vi "AddChannel.vi"(0 "VIRef":refnum<vi>[](array[refnum]), 1 "Name":string="172.16.21.19", 3 "SetCurrent":dbl format="%#.2g", 5 "ADRESS":string[](array[string]), 7 "error in (no error)":errorcluster, 9 "NAME":string[](array[string]), 11 "Address":string="172.16.21.19", 12 "SetVoltage":dbl format="%#.2g") -> (4 "NumRows":i32, 6 "NAMEOut":string[](array[string]), 8 "error out":errorcluster, 10 "ADRESSOut":string[](array[string]), 15 "VIRefOut":refnum<vi>[](array[refnum]))   [LabVIEW 2013]
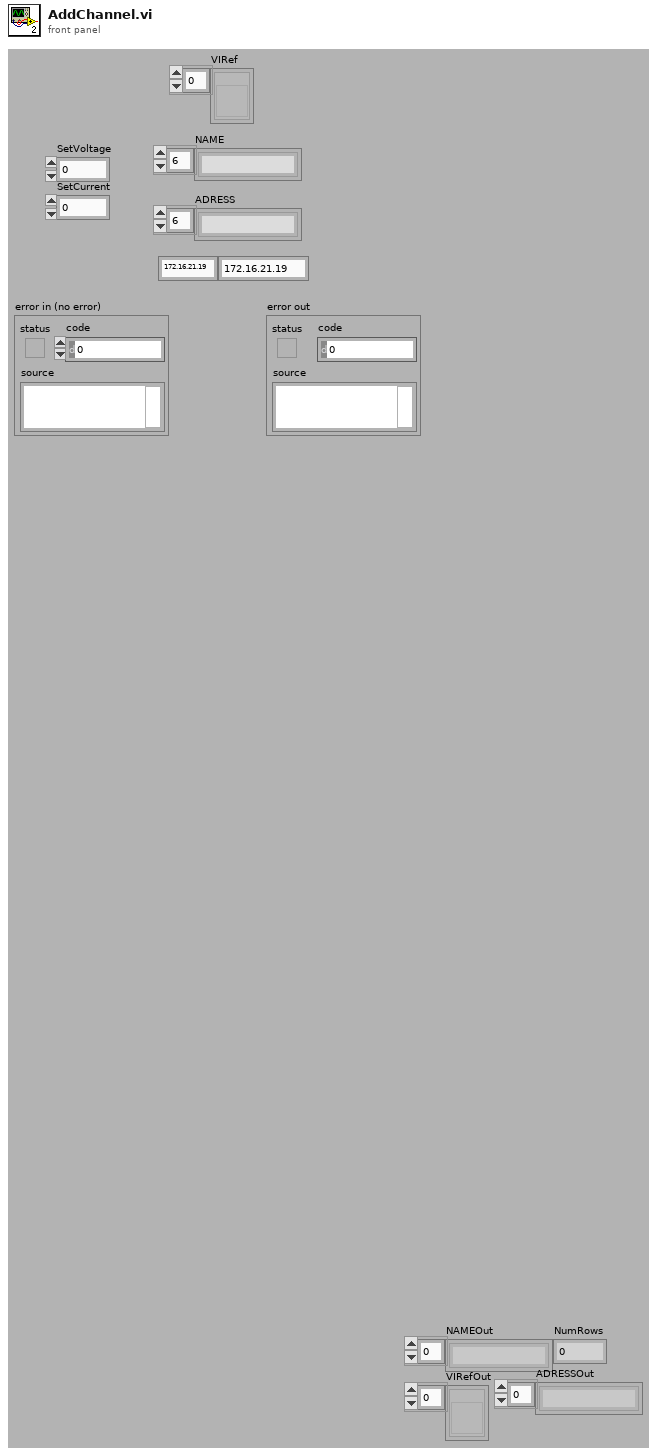
[diagram p1: front panel]
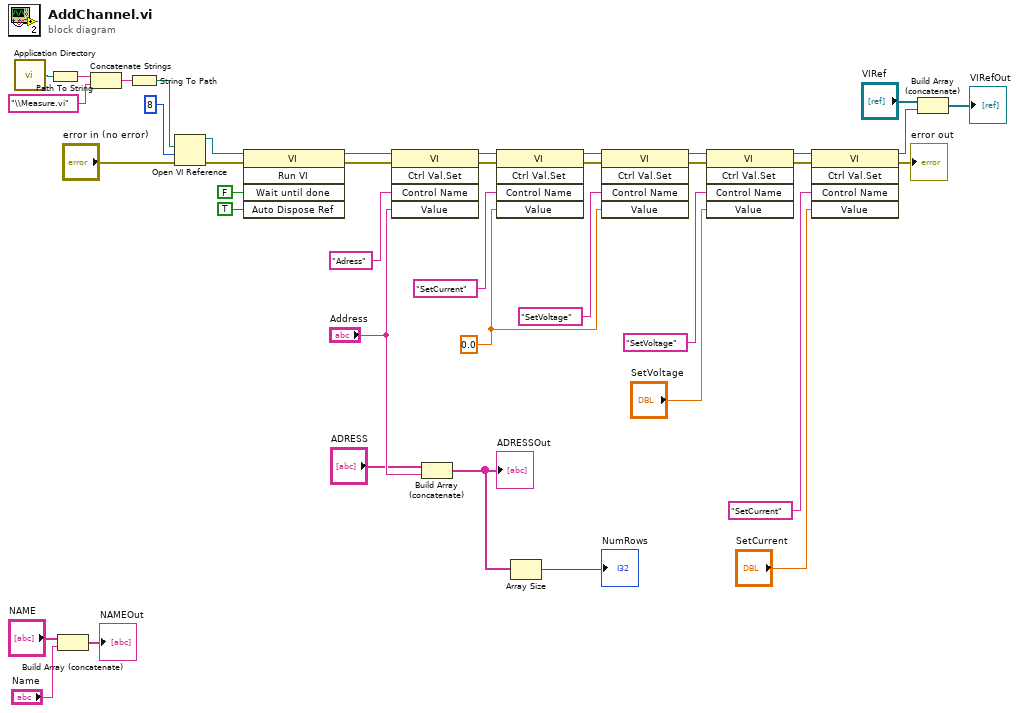
[diagram p0: block diagram]
diagram:
  w20 = 0.0 ("SetCurrent")
  n1 = call <vilib>:"Application Directory.vi"() -> ("Application Directory"=w1:path)
  n2 = Path To String(path=w1) -> (string=w5:string)
  n3 = Build Array (concatenate)("NAME", "Name") -> (→"NAMEOut":string[])
  n4 = Concatenate Strings(w5, "\\Measure.vi" ("string")) -> (w3:string)
  n5 = String To Path(string=w3) -> (path=w2:path)
  n6 = Open VI Reference(vi path=w2, options=8, error in (no error)="error in (no error)") -> (vi reference=w36:refnum<vi>, error out=w39:errorcluster)  [unwired: 1 in, 2 out]
  n7 = invoke class="VI" method="Run VI"(reference=w36, error in=w39, "Wait until done"=FALSE ("Wait Until Done"), "Auto Dispose Ref"=TRUE ("Auto Dispose Reference")) -> (reference out=w33:refnum<vi>, error out=w23:errorcluster)  [unwired: 1 in, 3 out]
  n8 = invoke class="VI" method="Ctrl Val.Set"(reference=w33, error in=w23, "Control Name"="Adress", "Value"="Address") -> (reference out=w25:refnum<vi>, error out=w22:errorcluster)  [unwired: 1 in, 3 out]
  n9 = Build Array (concatenate)("ADRESS", "Address") -> (w31:string[])
  "ADRESSOut" <- w31
  n10 = invoke class="VI" method="Ctrl Val.Set"(reference=w25, error in=w22, "Control Name"="SetCurrent", "Value"=w20) -> (reference out=w24:refnum<vi>, error out=w21:errorcluster)  [unwired: 1 in, 3 out]
  n11 = Array Size(array=w31) -> (size(s)=→"NumRows":i32)
  n12 = invoke class="VI" method="Ctrl Val.Set"(reference=w24, error in=w21, "Control Name"="SetVoltage", "Value"=w20) -> (reference out=w15:refnum<vi>, error out=w14:errorcluster)  [unwired: 1 in, 3 out]
  n13 = invoke class="VI" method="Ctrl Val.Set"(reference=w15, error in=w14, "Control Name"="SetVoltage", "Value"="SetVoltage") -> (reference out=w19:refnum<vi>, error out=w18:errorcluster)  [unwired: 1 in, 3 out]
  n14 = invoke class="VI" method="Ctrl Val.Set"(reference=w19, error in=w18, "Control Name"="SetCurrent", "Value"="SetCurrent") -> (reference out=w11:refnum<vi>, error out=→"error out":errorcluster)  [unwired: 1 in, 3 out]
  n15 = Build Array (concatenate)("VIRef", w11) -> (→"VIRefOut":refnum<vi>[])
